vi "Calibrate In Ear.vi"(11 "State":T1) -> (0 "error out":errorcluster)   [LabVIEW 2020]
uses:
  epl-vi-lib/Utility VIs/Conversion VIs/Create Waveform Cluster (2D).vi
  Instance           1 24Saved   Calibrate In Ear .vi
  epl-vi-lib/Utility VIs/Type Defs/Speaker ring.ctl
  Type Defs/Cal Stimulus.ctl
  Type Defs/ACal-In Ear Parameters.ctl
  Type Defs/ACal-Multiband Parameters.ctl
  epl-vi-lib/Utility VIs/Math VIs/FFT x(t) to dB,Degrees (2D).vi
  epl-vi-lib/Utility VIs/File IO VIs/Configuration File Wrapper VIs/Config-Read Key (Boolean).vi
  cfts/LV Source/CFTS Main Panel SubVIs/CFTS-Experiment State.ctl
  epl-vi-lib/Utility VIs/Buttons/KCheckmarkBoolean 2.ctl
panel:
  in  "Speaker":T2
  in  "mic gain":dbl caption="Probe Mic Gain (dB)"
  in  "Stimulus":T3={"Min Freq (Hz)"=1000.0, "Max Freq (Hz)"=50000.0, "Freq Step (Hz)"=50.0, "Waveform"=0, "Attenuation (dB)"=30.0, "Sample Rate (Hz)"=100000.0} {"Waveform" items=["Chirp"]}
  out "Stimulus graph":cluster{i32, dbl, dbl[]}(graph)={0, 0.01, []}
  in  "Averages":i32=128
  in  "Return":bool
  in  "START":bool
  in  "STOP":bool
  out "Path":path
  in  "Data tab":enum32{"Raw", "Calibration"}(tab)
  out "Mic signals":cluster{"offset":dbl, "dx":dbl, "Y":dbl[][]}(graph)
  out "Mic mag":cluster{"offset":dbl, "dx":dbl, "Y":dbl[][]}(graph)
  out "Acquired":i32=256
  in  "Clear":bool
  in  "Load":bool
  in  "Show all":bool
  in  "Last N":bool
  out "ASTF":cluster{"Frequency":dbl[], "Frequency":dbl[]}[](graph)
  in  "Plot Max SPL":T4=TRUE
  in  "result":cluster{"Path":path, "error ":errorcluster}
  out "ASTF phase":cluster{"Frequency":dbl[], "Frequency":dbl[]}[](graph)
  out "Mic phase graph":cluster{"offset":dbl, "dx":dbl, "Y":dbl[][]}(graph)
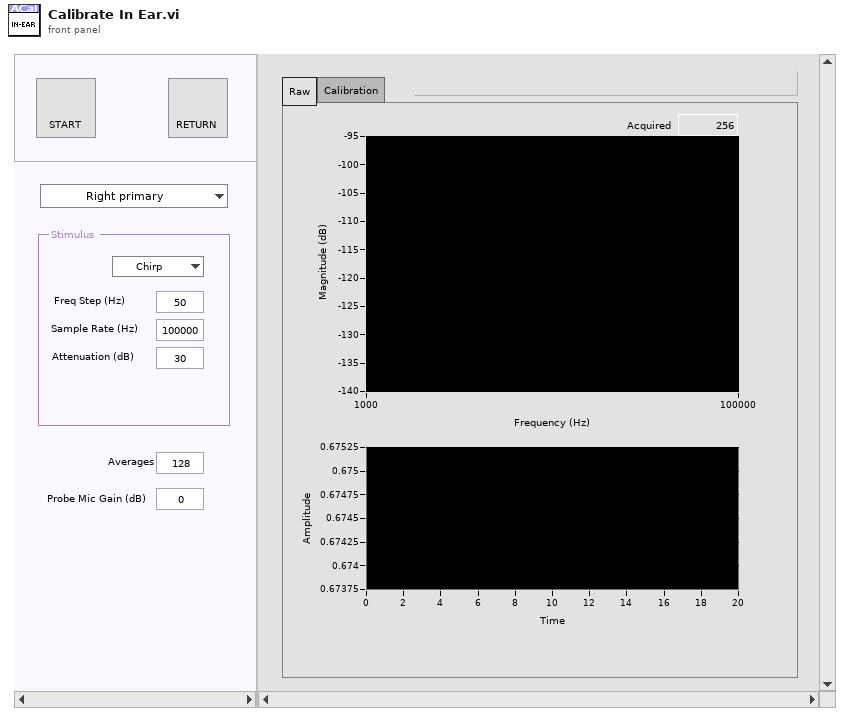
[diagram p1: front panel]
types:
  T1 = typedef "CFTS-Experiment State.ctl" = cluster{"Experimenter":string, "Number":u32, "Right":string, "Left":string, "Data Folder":path, "State File":path, "Version Info":string, "End Exposure Time":dbl, "Exposure Duration":string, "Run #":cluster{"CAP":i16, "ABR":i16, "DP":i16, "VsEP":i16, "MeasSeq":i16, "SubSeq":i16, "SFOAE":i16}}
  T2 = typedef "Speaker ring.ctl" = enum16{"Right primary", "Right secondary", "Left primary", "Left secondary"}
  T3 = cluster{"Min Freq (Hz)":dbl, "Max Freq (Hz)":dbl, "Freq Step (Hz)":dbl, "Waveform":u16, "Attenuation (dB)":dbl, "Sample Rate (Hz)":dbl}
  T4 = typedef "KCheckmarkBoolean 2.ctl" = bool
  T5 = typedef "ACal-In Ear Parameters.ctl" = cluster{"Speaker":T2, "Stimulus":T6, "Averages":i32, "Left gain":dbl, "Right gain":dbl, "plot max":bool, "smooth override":bool, "Weighted":T7, "Max Vmic":dbl}
  T6 = typedef "Cal Stimulus.ctl" = cluster{"Min Freq (Hz)":dbl, "Max Freq (Hz)":dbl, "Freq Step (Hz)":dbl, "Waveform":enum16{"Chirp", "Weighted"}, "Attenuation (dB)":dbl, "Sample Rate (Hz)":dbl}
  T7 = typedef "ACal-Multiband Parameters.ctl" = cluster{"Folder":path, "Fmin":dbl, "Fmax":dbl, "Max range":dbl, "WF":u16}
  T8 = typedef "Cal-Smoothing Parameters.ctl" = cluster{"Method":enum16{"None", "Moving average", "Loess"}, "MA":cluster{"Iterations":i32, "Length":i32}, "Loess":cluster{"Length":i32, "Type":enum16{"Linear", "Quadratic"}, "Robust":bool}}
  T9 = cluster{"new file path":path, "error out":errorcluster}
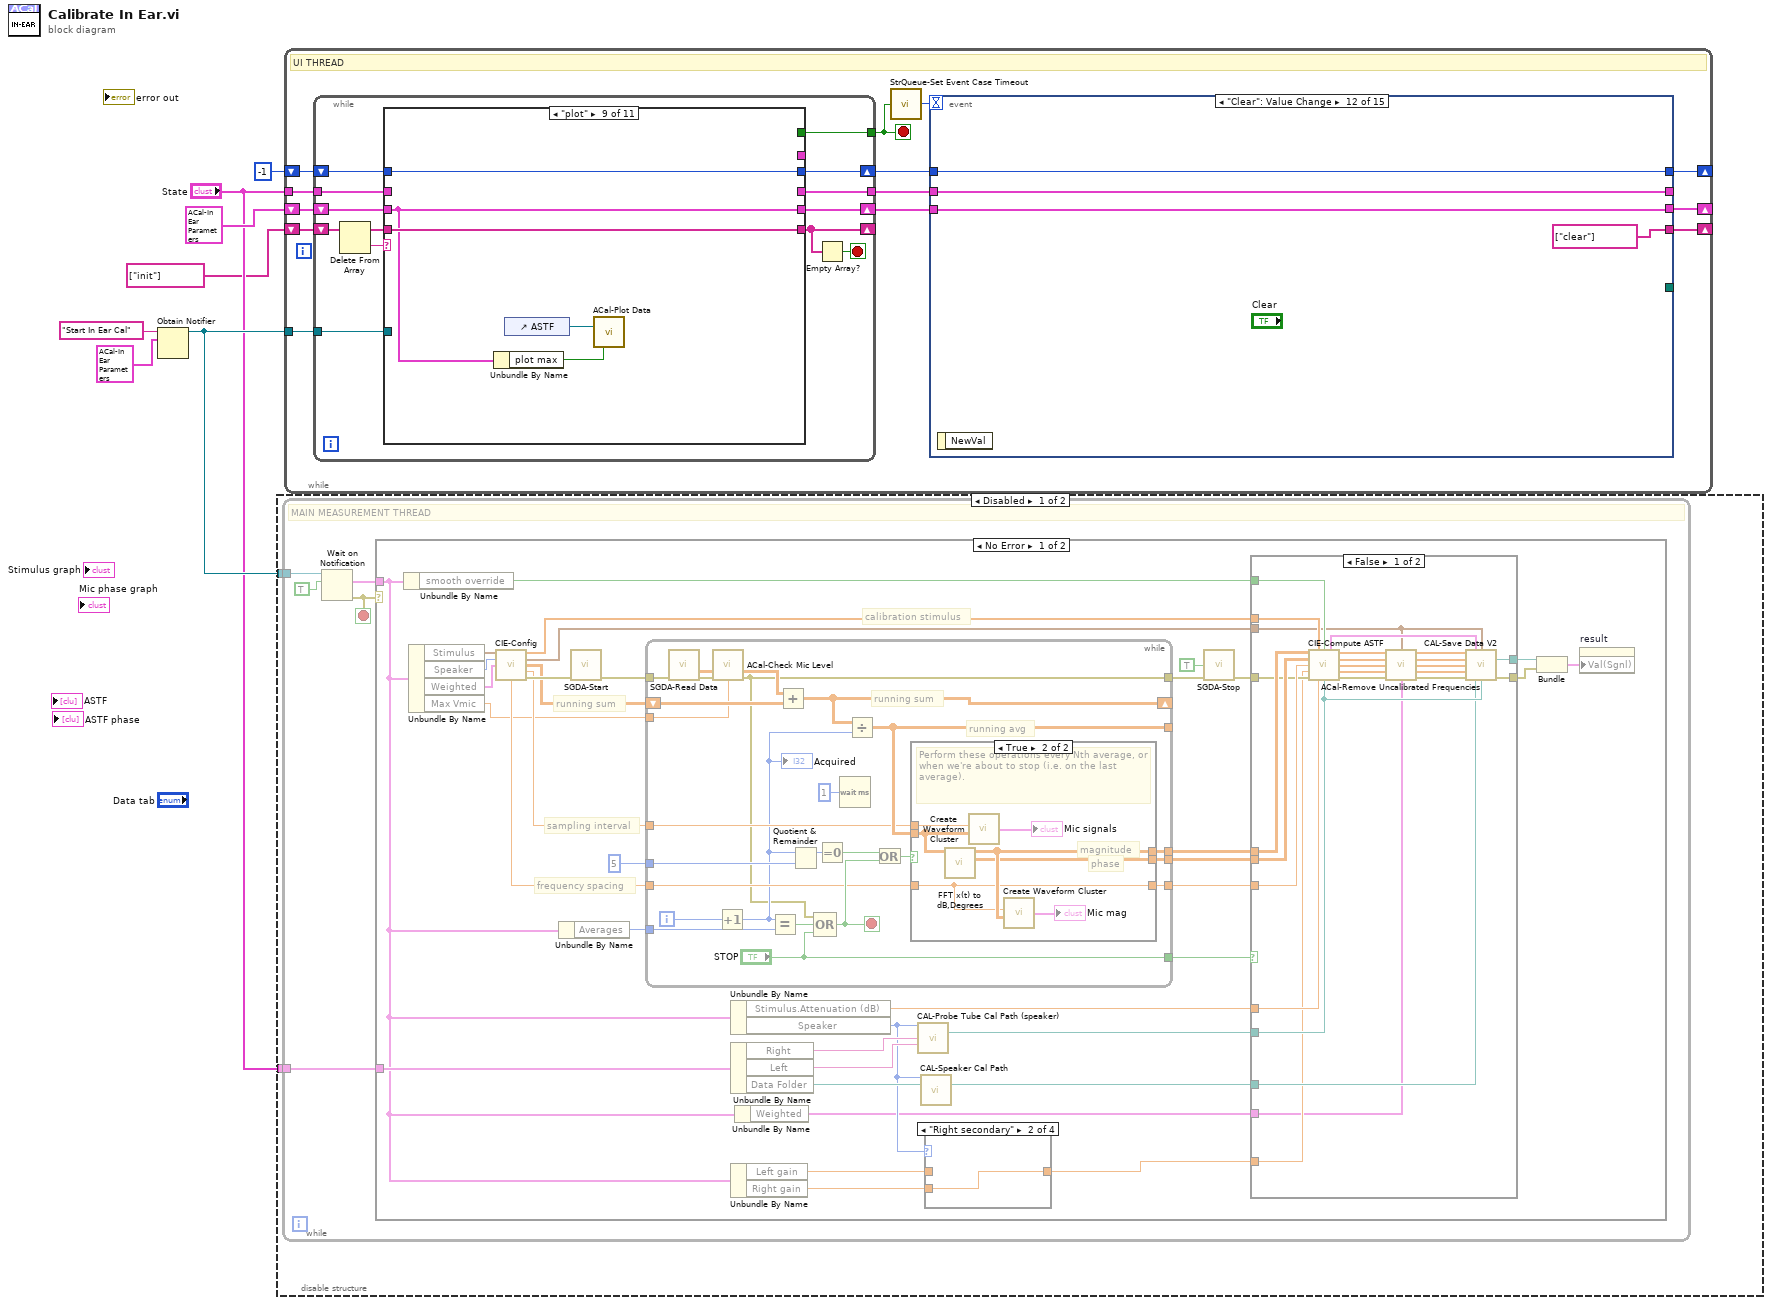
[diagram p0: block diagram]
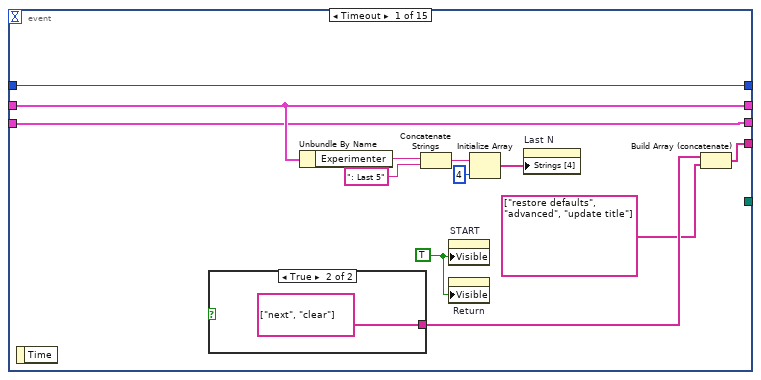
[diagram p9: hidden frame]
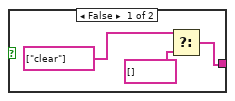
[diagram p10: hidden frame]
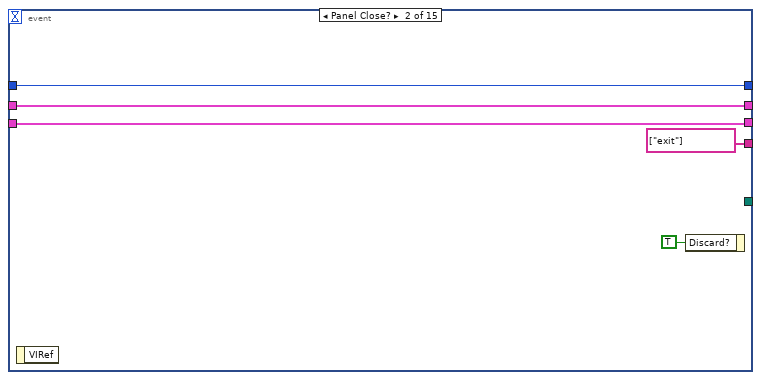
[diagram p11: hidden frame]
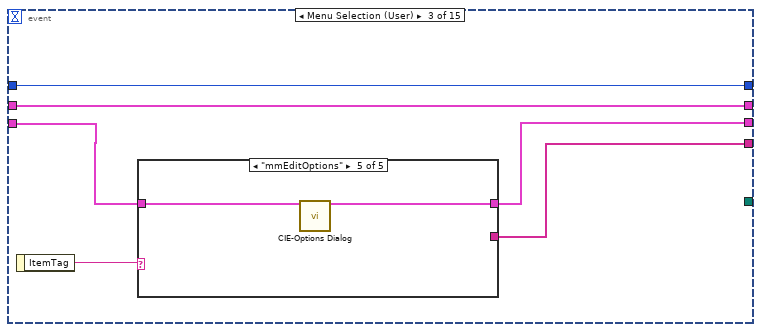
[diagram p12: hidden frame]
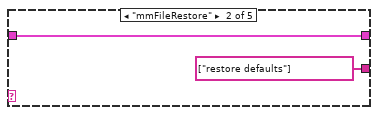
[diagram p14: hidden frame]
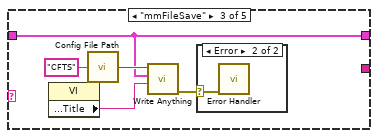
[diagram p15: hidden frame]
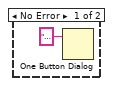
[diagram p16: hidden frame]
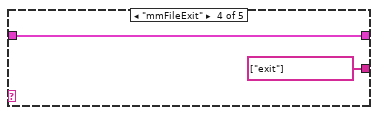
[diagram p17: hidden frame]
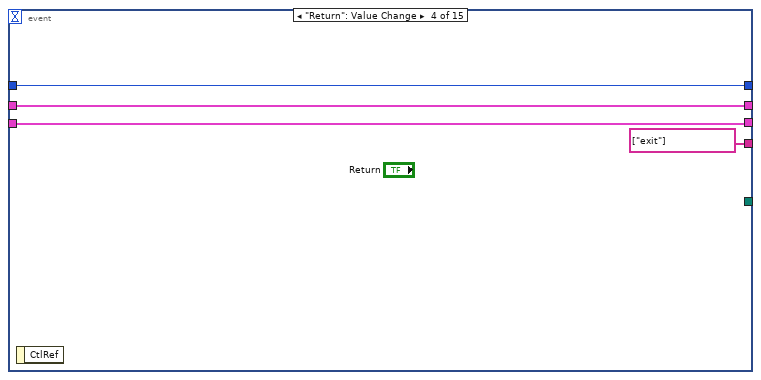
[diagram p18: hidden frame]
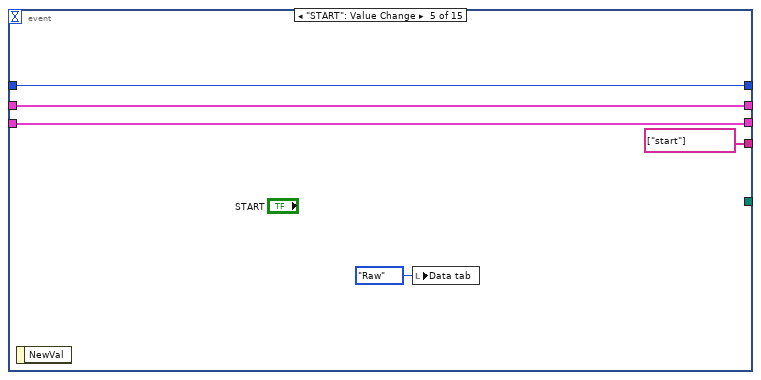
[diagram p19: hidden frame]
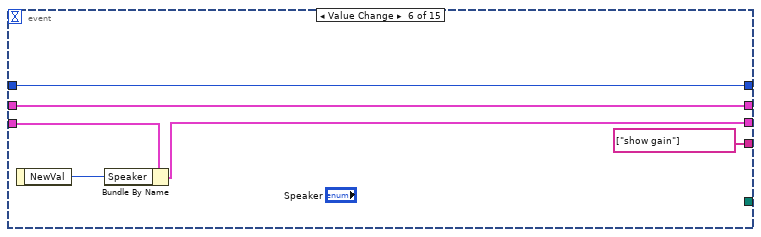
[diagram p20: hidden frame]
diagram:
  n1 = Obtain Notifier(name (unnamed)="Start In Ear Cal", notification data type=T5 {"Speaker"=enum."Right primary", "Stimulus"={"Min Freq (Hz)"=50.0, "Max Freq (Hz)"=50000.0, "Freq Step (Hz)"=50.0, "Waveform"=enum."Chirp", "Attenuation (dB)"=20.0, "Sample Rate (Hz)"=100000.0}, "Averages"=512, "Left gain"=40.0, "Right gain"=40.0, "plot max"=TRUE, "smooth override"=FALSE, "Weighted"={"Folder"=path "", "Fmin"=0.0, "Fmax"=0.0, "Max range"=0.0, "WF"=0}, "Max Vmic"=0.0} ("Params")) -> (notifier out=w7:refnum<notifier>)  [unwired: 2 in, 2 out]
  n2 = disable-structure shown="Disabled" {
    disable-tunnel: w7 -> [w9 _]
    disable-tunnel: "State" -> [w8 _]
    frame Disabled {
      n3 = while {
        tunnel: w9 -> [w14]
        tunnel: w8 -> [w12]
        stop <- w13 stop-if-true
        # "MAIN MEASUREMENT THREAD"
        n4 = Wait on Notification(notifier=w14, ignore previous (F)=TRUE) -> (notification=w11:T5, error out=w13:errorcluster)  [unwired: 2 in, 2 out]
        n5 = case shown="No Error" w13 {
          tunnel: w12 -> [w33 _]
          tunnel: w11 -> [w18 _]
          frame No Error {
            # "calibration stimulus"
            # "frequency spacing"
            # "sampling interval"
            # "running sum"
            n6 = Unbundle By Name(w18) -> ("smooth override"=w29:bool)
            n7 = Unbundle By Name(w18) -> ("Stimulus"=w32:T6, "Speaker"=w31:T2, "Weighted"=w19:T7, "Max Vmic"=w16:dbl)
            n8 = call "CIE-Config.vi"("Cal Stimulus"=w32, "Speaker"=w31, "Weighted"=w19) -> ("Stimulus"=w44:dbl[], "Cal Spec Out"=w35:T6, "Mic Avg"=w50:dbl[][], "dt (ms)"=w48:dbl, "df (Hz)"=w49:dbl, "error out"=w51:errorcluster)  [unwired: 6 in, 1 out]
            n9 = Unbundle By Name(w18) -> ("Averages"=w30:i32)
            n10 = call "SGDA-Start.vi"("error in (no error)"=w51) -> ("error out"=w43:errorcluster)  [unwired: 6 in]
            n11 = while {
              tunnel: w43 -> [w106]
              tunnel: [w82] -> w42
              tunnel: w30 -> [w103]
              shift-right: [w101] -> _
              shift-left: w50 -> [w102]
              tunnel: [w100] -> _
              tunnel: 5 -> [w99]
              tunnel: w49 -> [w94]
              tunnel: [w93] -> w47
              tunnel: [w92] -> w46
              tunnel: w48 -> [w91]
              tunnel: [w90] -> w45
              tunnel: ["STOP"] -> w27
              tunnel: w16 -> [w83]
              i -> [w105]
              stop <- w95 stop-if-true
              # "running avg"
              # "running sum"
              n12 = call "SGDA-Read Data.vi"("error in (no error)"=w106) -> ("AI Waveforms"=w85:dbl[][], "error out"=w86:errorcluster)  [unwired: 13 in]
              n13 = call "ACal-Check Mic Level.vi"("AI Waveforms in"=w85, "error in (no error)"=w86, "Max Vmic"=w83) -> ("AI Waveforms out"=w84:dbl[][], "error out"=w82:errorcluster)  [unwired: 11 in]
              n14 = Increment(x=w105) -> (x+1=w89:i32)
              "Acquired" <- w89
              n15 = Equal?(x=w89, y=w103) -> (x = y?=w104:bool)
              n16 = Add(x=w84, y=w102) -> (x+y=w101:dbl[][])
              n17 = Quotient & Remainder(x=w89, y=w99) -> (x-y*floor(x/y)=w98:i32)  [unwired: 1 out]
              n18 = Compound Arithmetic op=OR(w82, w104, "STOP") -> (w95:bool)
              n19 = Equal To 0?(x=w98) -> (x = 0?=w96:bool)
              n20 = Wait (ms)(milliseconds to wait=u32 1) -> ()  [unwired: 1 out]
              n21 = Divide(x=w101, y=w89) -> (x/y=w100:dbl[][])
              n22 = Or(x=w96, y=w95) -> (x .or. y?=w97:bool)
              n23 = case shown="True" w97 {
                tunnel: w100 -> [_ w110]
                tunnel: w94 -> [_ w107]
                tunnel: [_ w112] -> w93
                tunnel: [_ w111] -> w92
                tunnel: w91 -> [_ w109]
                tunnel: [_ w107] -> w90
                frame False {
                }
                frame True {
                  # "phase"
                  # "magnitude"
                  # "Perform these operations every Nth average, or when we're about to stop (i.e. on the last average)."
                  n24 = call-poly "FFT x(t) to dB,Degrees.vi"("X(t)"=w110) -> ("+Freq Phase of FFT (degrees)"=w111:dbl[][], "+Freq. Mag of FFT (dB rms)"=w112:dbl[][])  [unwired: 9 in]
                  n25 = call-poly "Create Waveform Cluster.vi"("dx"=w109, "Array"=w110) -> ("waveform cluster"=→"Mic signals":cluster{"offset":dbl, "dx":dbl, "Y":dbl[][]})  [unwired: 3 in]
                  n26 = call-poly "Create Waveform Cluster.vi"("dx"=w107, "Array"=w112) -> ("waveform cluster"=→"Mic mag":cluster{"offset":dbl, "dx":dbl, "Y":dbl[][]})  [unwired: 3 in]
                }
              }
            }
            n27 = Unbundle By Name(w18) -> ("Stimulus.Attenuation (dB)"=w28:dbl, "Speaker"=w26:T2)
            n28 = Unbundle By Name(w33) -> ("Right"=w40:string, "Left"=w39:string, "Data Folder"=w38:path)
            n29 = Unbundle By Name(w18) -> ("Left gain"=w25:dbl, "Right gain"=w23:dbl)
            n30 = Unbundle By Name(w18) -> ("Weighted"=w17:T7)
            n31 = call "CAL-Probe Tube Cal Path (speaker).vi"("Speaker"=w26, "Right"=w40, "Left"=w39) -> ("Probe Tube Cal Path"=w37:path)  [unwired: 11 in, 1 out]
            n32 = call "CAL-Speaker Cal Path.vi"("Speaker"=w26, "Data Folder"=w38) -> ("Cal Path"=w34:path)  [unwired: 12 in, 1 out]
            n33 = case shown="\"Right secondary\"" w26 {
              tunnel: w25 -> [_ _ w54 w55]
              tunnel: [w52 w53 w54 w55] -> w24
              tunnel: w23 -> [w52 w53 _ _]
              frame "Right primary", Default {
              }
              frame "Right secondary" {
              }
              frame "Left secondary" {
              }
              frame "Left primary" {
              }
            }
            n34 = call "SGDA-Stop.vi"("Clear ActiveX (F)"=TRUE, "error in (no error)"=w42) -> ("error out"=w36:errorcluster)  [unwired: 13 in]
            n35 = case shown="False" w27 {
              tunnel: w47 -> [w80 _]
              tunnel: w46 -> [w79 _]
              tunnel: w45 -> [w78 _]
              tunnel: w44 -> [w77 _]
              tunnel: w37 -> [w76 _]
              tunnel: w36 -> [w75 w81]
              tunnel: w35 -> [w57 _]
              tunnel: w34 -> [w73 _]
              tunnel: w29 -> [w72 _]
              tunnel: w28 -> [w71 _]
              tunnel: [w70 w81] -> w21
              tunnel: [w69 _] -> w22
              tunnel: w24 -> [w68 _]
              tunnel: w17 -> [w56 _]
              frame False {
                n36 = call "CIE-Compute ASTF.vi"("Mag"=w80, "Stimulus"=w77, "Force no smoothing?"=w72, "Phase"=w79, "df (Hz)"=w78, "Probe Mic Gain (dB)"=w68, "error in (no error)"=w75, "Attenuation (dB)"=w71, "Probe Tube Path"=w76) -> ("Smooth Params"=w74:T8, "ASTF Mag"=w59:dbl[], "ASTF Phase"=w60:dbl[], "Frequency"=w63:dbl[], "Unsmoothed Mag"=w64:dbl[], "error out"=w67:errorcluster)  [unwired: 1 in]
                n37 = call "ACal-Remove Uncalibrated Frequencies.vi"("ASTF Mag in"=w59, "Cal Spec Out"=w57, "ASTF Phase in"=w60, "Frequency in"=w63, "Unsmoothed Mag in"=w64, "error in (no error)"=w67, "Weighted"=w56) -> ("ASTF Mag out"=w58:dbl[], "ASTF Phase out"=w61:dbl[], "Frequency out"=w62:dbl[], "Unsmoothed Mag out"=w65:dbl[], "error out"=w66:errorcluster)  [unwired: 4 in]
                n38 = call "CAL-Save Data V2.vi"("Mag"=w58, "Smooth Params"=w74, "Cal Stimulus"=w57, "Phase"=w61, "Frequency"=w62, "Unsmoothed Mag"=w65, "error in (no error)"=w66, "path"=w73, "Probe Tube File"=w76) -> ("new file path"=w69:path, "error out"=w70:errorcluster)  [unwired: 5 in]
              }
              frame True {
              }
            }
            n39 = Bundle("new file path"=w22, "error out"=w21) -> (w20:T9)  [unwired: 1 in]
            n40 = property on="result" class="Clust (strict)"("Val(Sgnl)"=w20) -> ()  [unwired: 2 in, 2 out]
          }
          frame Error {
          }
        }
      }
    }
    frame Enabled {
    }
  }
  n41 = while {
    tunnel: w7 -> [w119]
    shift-right: [w114] -> _
    shift-left: -1 -> [w126]
    tunnel: "State" -> [w125]
    shift-right: [w115] -> _
    shift-left: T5 {"Speaker"=enum."Right primary", "Stimulus"={"Min Freq (Hz)"=50.0, "Max Freq (Hz)"=50000.0, "Freq Step (Hz)"=50.0, "Waveform"=enum."Chirp", "Attenuation (dB)"=20.0, "Sample Rate (Hz)"=100000.0}, "Averages"=512, "Left gain"=40.0, "Right gain"=40.0, "plot max"=TRUE, "smooth override"=FALSE, "Weighted"={"Folder"=path "C:/Data", "Fmin"=3000.0, "Fmax"=45000.0, "Max range"=25.0, "WF"=0}, "Max Vmic"=0.0} ("Params") -> [w124]
    shift-right: [w122] -> _
    shift-left: string[] ["init"] ("t") -> [w121]
    stop <- w117 stop-if-true
    # "UI THREAD"
    n42 = while {
      shift-right: [w261] -> w120
      shift-left: w124 -> [w262]
      shift-right: [w260] -> w123
      shift-left: w126 -> [w263]
      shift-right: [w256] -> _
      shift-left: w121 -> [w258]
      tunnel: w119 -> [w254]
      tunnel: [w253] -> w117
      tunnel: w125 -> [w252]
      tunnel: [w251] -> w116
      stop <- w255 stop-if-true
      n43 = Delete From Array(array=w258) -> (deleted portion=w257:string, array with subset deleted=w259:string[])  [unwired: 2 in]
      n44 = case shown="\"plot\"" w257 {
        tunnel: w263 -> [w266 w271 w277 w288 w299 w315 w331 w338 w345 w350 w361]
        tunnel: [w266 w271 w277 w288 w299 w315 w331 w338 w345 w350 w361] -> w260
        tunnel: w262 -> [w265 w270 w276 w287 w298 w310 w329 w336 w343 w346 w355]
        tunnel: [w265 w270 w276 w287 w298 w309 w329 w336 w343 w346 w354] -> w261
        tunnel: w259 -> [w264 w269 w275 w286 w297 w314 w330 w337 w344 w347 w353]
        tunnel: [w264 w269 w275 w286 w297 w308 w324 w337 w344 w347 w351] -> w256
        tunnel: w254 -> [_ _ w274 _ _ _ _ _ _ w348 _]
        tunnel: [_ _ TRUE _ _ _ _ _ _ _ w358] -> w253
        tunnel: w252 -> [_ _ w272 w279 _ _ _ _ _ _ _]
        tunnel: [_ _ _ _ w293 _ _ _ _ _ w352] -> _
        tunnel: [_ _ w272 _ _ _ _ _ _ _ _] -> w251
        frame "", Default {
        }
        frame "clear" {
          w268 = cluster{"Frequency":dbl[], "Frequency":dbl[]}[] [] ("ASTF mag")
          n45 = property on="ASTF phase" class="XYGraph (strict)"("Value"=w268) -> ()  [unwired: 2 in, 2 out]
          n46 = property on="ASTF" class="XYGraph (strict)"("Legend Visible"=FALSE ("Legend:Visible"), "Value"=w268) -> ()  [unwired: 2 in, 2 out]
        }
        frame "exit" {
          n47 = Release Notifier(notifier=w274) -> ()  [unwired: 2 in, 3 out]
        }
        frame "update title" {
          n48 = Unbundle By Name(w279) -> ("Experimenter"=w278:string)
          n49 = control-ref of="This VI"() -> (w280:refnum<vi>)
          n50 = call "CFTS-Is Advanced User.vi"("Experimenter"=w278) -> ("Advanced user"=w283:bool)
          n51 = call "Config File Path.vi"("AppName"="CFTS") -> ("Default config file name"=w281:path)
          n52 = Select(t=w278, s=w283, f="") -> (s? t:f=w285:string)
          n53 = call "Append User ID To Section Label.vi"("VI reference"=w280, "Path (dialog)"=w281, "User"=w285) -> ()  [unwired: 9 in, 4 out]
        }
        frame "advanced" {
          n54 = call "PXI-Connections File Path.vi"() -> ("Path"=w294:path)  [unwired: 1 in]
          n55 = call-poly "Config-Read Key.vi"("configuration file path"=w294, "key"="Advanced in-ear", "default"=FALSE) -> ("value"=w292:bool)  [unwired: 9 in, 3 out]
          n56 = case shown="True" w292 {
            tunnel: "Chirp" ("key") -> [w301 w304]
            tunnel: "Weighted" ("key") -> [_ w303]
            tunnel: [w300 w302] -> w289
            frame False {
              n57 = Build Array(w301) -> (w300:string[])
            }
            frame True {
              n58 = Build Array(w304, w303) -> (w302:string[])
            }
          }
          n59 = Bundle By Name("advanced"=w292) -> (w293:cluster{})  [unwired: 1 in]
          n60 = property on="Waveform" class="Ring (strict)"("Strings []"=w289) -> ()  [unwired: 2 in, 2 out]
        }
        frame "restore defaults" {
          n61 = property class="VI"() -> ("Front Panel.Title"=w306:string)  [unwired: 2 in, 2 out]
          n62 = call "Config File Path.vi"("AppName"="CFTS") -> ("Default config file name"=w305:path)
          n63 = call "Read Anything.vi"("Type of Anything"=w310, "Section Name (Name of \"Type of Anything\")"=w306, "Path (dialog)"=w305) -> ("Found?"=w312:bool, "Anything"=w311:variant)  [unwired: 6 in, 1 out]
          n64 = case shown="False" w312 {
            tunnel: w311 -> [_ w321]
            tunnel: w310 -> [w318 w320]
            tunnel: [w317 w319] -> w309
            tunnel: w306 -> [w316 _]
            frame False {
              n65 = call "ACal-Update In Ear Parameters.vi"("Params in"=w318, "Section"=w316) -> ("Params out"=w317:T5)  [unwired: 13 in]
            }
            frame True {
              n66 = Variant To Data(type=w320, Variant=w321) -> (data=w319:T5)  [unwired: 1 in, 1 out]
            }
          }
          n67 = Build Array (concatenate)(w314, "show params") -> (w308:string[])
        }
        frame "show params" {
          n68 = Unbundle By Name(w329) -> ("Speaker"=w328:T2, "Stimulus"=w327:T6, "Averages"=w326:i32, "plot max"=w325:bool)
          n69 = local write "Speaker"(w328) -> ()
          n70 = local write "Stimulus"(w327) -> ()
          n71 = local write "Averages"(w326) -> ()
          n72 = local write "Plot Max SPL"(w325) -> ()
          n73 = Build Array (concatenate)(w330, "show gain", "show wf") -> (w324:string[])
        }
        frame "show gain" {
          n74 = Unbundle By Name(w336) -> ("Speaker"=w334:T2, "Left gain"=w333:dbl, "Right gain"=w332:dbl)
          n75 = case shown="\"Right primary\", \"Right secondary\"" w334 {
            tunnel: w333 -> [w339 _]
            tunnel: w332 -> [_ w340]
            tunnel: [w339 w340] -> w335
            frame "Left primary", Default {
            }
            frame "Right primary", "Right secondary" {
            }
          }
          n76 = local write "mic gain"(w335) -> ()
        }
        frame "plot" {
          n77 = Unbundle By Name(w343) -> ("plot max"=w342:bool)
          n78 = control-ref of="ASTF"() -> (w341:refnum<vi>)
          n79 = call "ACal-Plot Data.vi"("Mag graph"=w341, "Plot max"=w342) -> ()  [unwired: 12 in, 2 out]
        }
        frame "start" {
          w349 = FALSE
          n80 = Send Notification(notification=w346, notifier=w348) -> ()  [unwired: 1 in, 2 out]
          n81 = property on="Return" class="Bool"("Visible"=w349) -> ()  [unwired: 2 in, 2 out]
          n82 = property on="START" class="Bool"("Visible"=w349) -> ()  [unwired: 2 in, 2 out]
        }
        frame "next" {
          w357 = T2[] [enum."Right primary", enum."Right secondary", enum."Left primary", enum."Left secondary"] items=["Right primary", "Right secondary", "Left primary", "Left secondary"]
          n83 = Unbundle By Name() -> ()  [unwired: 1 in, 1 out]
          n84 = Array Size(array=w357) -> (size(s)=w360:i32)
          n85 = Increment() -> (x+1=w356:dbl)  [unwired: 1 in]
          n86 = Less?(x=w356, y=w360) -> (x < y?=w359:bool)
          n87 = case shown="True" w359 {
            tunnel: [TRUE _] -> w358
            tunnel: w357 -> [_ w371]
            tunnel: w356 -> [_ w367]
            tunnel: w355 -> [w363 w370]
            tunnel: [w363 w368] -> w354
            tunnel: [w362 string[] ["start"]] -> w351
            tunnel: w353 -> [w362 _]
            tunnel: [_ w366] -> w352
            frame False {
            }
            frame True {
              n88 = Index Array(array=w371, index=w367) -> (element=w369:T2)
              n89 = Bundle By Name(cluster=w370, "Speaker"=w369) -> (w368:T5)
              n90 = local write "Speaker"(w369) -> ()
              n91 = Bundle By Name("next"=w367) -> (w366:cluster{})  [unwired: 1 in]
            }
          }
        }
      }
      n92 = Empty Array?(array=w256) -> (empty?=w255:bool)
    }
    n93 = call "StrQueue-Set Event Case Timeout.vi"("Quit"=w117) -> ("timeout"=w118:i32)  [unwired: 14 in]
    n94 = event shown="[11] \"Clear\": Value Change" {
      selector: _ -> [_ _ _ _ _ _ _ _ _ _ _ _ _ _ _]
      dyn-events: _ -> [_ _ _ _ _ _ _ _ _ _ _ _ _ _ _]
      timeout: w118 -> [_ _ _ _ _ _ _ _ _ _ _ _ _ _ _]
      tunnel: w123 -> [w132 w146 w153 w171 w176 w182 w186 w191 w198 w209 w218 w228 w233 w244 w249]
      tunnel: [w132 w146 w153 w171 w176 w182 w186 w191 w198 w209 w218 w228 w233 w244 w249] -> w114
      tunnel: w120 -> [w127 w143 w149 w169 w173 w179 w185 w190 w194 w206 w210 w225 w232 w242 w246]
      tunnel: [w127 w143 w151 w169 w173 w178 w184 w189 w193 w205 w210 w225 w232 w242 w246] -> w115
      tunnel: [w130 string[] ["exit"] w150 string[] ["exit"] string[] ["start"] string[] ["show gain"] _ _ _ _ w214 string[] ["clear"] w230 _ _] -> w122
      tunnel: [w128 w144 w148 w168 w172 w177 w183 w188 w195 w207 w211 w226 w229 w241 w247] -> _
      tunnel: [_ _ _ _ _ _ _ _ _ _ w216 _ w231 _ _] -> _
      tunnel: w116 -> [w128 w144 w148 w168 w172 w177 w183 w188 w195 w207 w211 w226 w229 w241 w247]
      event Timeout {
        w138 = TRUE ("Visible")
        n95 = event-data() -> ()  [unwired: 1 in, 1 out]
        n96 = case shown="True" {
          selector: _ -> [_ _]
          tunnel: [w140 string[] ["next", "clear"]] -> w131
          frame False {
            n97 = Select(t=string[] ["clear"], f=string[] []) -> (s? t:f=w140:string[])  [unwired: 1 in]
          }
          frame True {
          }
        }
        n98 = Unbundle By Name(w128) -> ("Experimenter"=w137:string)
        n99 = Concatenate Strings(w137, ": Last 5" ("string")) -> (w135:string)
        n100 = property on="START" class="Bool"("Visible"=w138) -> ()  [unwired: 2 in, 2 out]
        n101 = property on="Return" class="Bool"("Visible"=w138) -> ()  [unwired: 2 in, 2 out]
        n102 = Initialize Array(w135, 4 ("dimension size")) -> (w133:string[])
        n103 = property on="Last N" class="Bool"("Strings [4]"=w133) -> ()  [unwired: 2 in, 2 out]
        n104 = Build Array (concatenate)(w131, string[] ["restore defaults", "advanced", "update title"]) -> (w130:string[])
      }
      event Panel Close? {
        n105 = event-data() -> ()  [unwired: 1 in, 1 out]
        n106 = event-data("Discard?"=TRUE) -> ()  [unwired: 1 in, 1 out]
      }
      event Menu Selection (User) {
        n107 = event-data() -> ("ItemTag"=w152:string)  [unwired: 1 in]
        n108 = case shown="\"mmEditOptions\"" w152 {
          tunnel: w149 -> [w154 w156 w159 w165 w167]
          tunnel: [w154 w156 w159 w165 w166] -> w151
          tunnel: [_ string[] ["restore defaults"] _ string[] ["exit"] _] -> w150
          frame "", Default {
          }
          frame "mmFileRestore" {
          }
          frame "mmFileSave" {
            n109 = property class="VI"() -> ("Front Panel.Title"=w158:string)  [unwired: 2 in, 2 out]
            n110 = call "Config File Path.vi"("AppName"="CFTS") -> ("Default config file name"=w160:path)
            n111 = call "Write Anything.vi"("Section Name (Name of \"Anything\")"=w158, "Anything"=w159, "Path (dialog)"=w160) -> ("Error Out"=w157:errorcluster)  [unwired: 7 in, 1 out]
            n112 = case shown="Error" w157 {
              selector: w157 -> [_ w163]
              frame No Error {
                n113 = One Button Dialog(message="Defaults saved.") -> ()  [unwired: 1 in, 1 out]
              }
              frame Error {
                n114 = call "Error Handler.vi"("error in (no error)"=w163) -> ()  [unwired: 13 in, 2 out]
              }
            }
          }
          frame "mmFileExit" {
          }
          frame "mmEditOptions" {
            n115 = call "CIE-Options Dialog.vi"("Override smoothing"=w167) -> ("Override Out"=w166:T5)  [unwired: 13 in, 1 out]
          }
        }
      }
      event "Return": Value Change {
        n116 = event-data() -> ()  [unwired: 1 in, 1 out]
      }
      event "START": Value Change {
        n117 = event-data() -> ()  [unwired: 1 in, 1 out]
        n118 = local write "Data tab"(enum32{"Raw", "Calibration"}."Raw" ("Data tab")) -> ()
      }
      event Value Change {
        n119 = event-data() -> ("NewVal"=w180:T2)  [unwired: 1 in]
        n120 = Bundle By Name(cluster=w179, "Speaker"=w180) -> (w178:T5)
      }
      event "Stimulus": Value Change {
        n121 = event-data() -> ()  [unwired: 1 in, 1 out]
        n122 = Bundle By Name(cluster=w185, "Stimulus"="Stimulus") -> (w184:T5)
      }
      event "Averages": Value Change {
        n123 = event-data() -> ()  [unwired: 1 in, 1 out]
        n124 = Bundle By Name(cluster=w190, "Averages"="Averages") -> (w189:T5)
      }
      event "mic gain": Value Change {
        n125 = event-data() -> ()  [unwired: 1 in, 1 out]
        n126 = Unbundle By Name(w194) -> ("Speaker"=w196:T2)
        n127 = case shown="\"Left primary\", Default" w196 {
          tunnel: [w201 w204] -> w193
          tunnel: "mic gain" -> [w200 w203]
          tunnel: w194 -> [w199 w202]
          frame "Left primary", Default {
            n128 = Bundle By Name(cluster=w199, "Left gain"=w200) -> (w201:T5)
          }
          frame "Right primary", "Right secondary" {
            n129 = Bundle By Name(cluster=w202, "Right gain"=w203) -> (w204:T5)
          }
        }
      }
      event Value Change {
        n130 = event-data() -> ()  [unwired: 1 in, 1 out]
        n131 = Bundle By Name(cluster=w206, "plot max"="Plot Max SPL") -> (w205:T5)
      }
      event "result": Value Change {
        w215 = TRUE
        n132 = event-data() -> ("NewVal.Path"=w217:path, "NewVal.error"=w213:errorcluster)  [unwired: 1 in]
        n133 = call "Beeper.vi"() -> ()  [unwired: 5 in, 1 out]
        n134 = case shown="No Error" w213 {
          selector: w213 -> [_ w224]
          tunnel: w217 -> [w223 _]
          tunnel: [w223 _] -> w216
          tunnel: [w220 _] -> w214
          frame No Error {
            n135 = Empty String/Path?(string/path=w223) -> (empty?=w222:bool)
            n136 = Select(t=string[] [], s=w222, f=string[] ["plot"]) -> (s? t:f=w220:string[])
            "Path" <- w223
          }
          frame Error {
            n137 = call "Error Handler.vi"("error in (no error)"=w224) -> ()  [unwired: 13 in, 2 out]
          }
        }
        n138 = local write "Data tab"(enum32{"Raw", "Calibration"}."Calibration" ("Data tab")) -> ()
        n139 = property on="START" class="Bool"("Visible"=w215) -> ()  [unwired: 2 in, 2 out]
        n140 = property on="Return" class="Bool"("Visible"=w215) -> ()  [unwired: 2 in, 2 out]
      }
      event "Clear": Value Change {
        n141 = event-data() -> ()  [unwired: 1 in, 1 out]
      }
      event "Load": Value Change {
        n142 = event-data() -> ()  [unwired: 1 in, 1 out]
        n143 = Unbundle By Name(w232) -> ()  [unwired: 1 out]
        n144 = call "File Dialog"("pattern (all files)"="*.calib", "pattern label"="Calibration files") -> ("selected path"=w238:path, "cancelled"=w237:bool, "error out"=w236:errorcluster)  [unwired: 10 in, 1 out]
        n145 = case shown="False" w237 {
          tunnel: w238 -> [w240 _]
          tunnel: w236 -> [_ _]
          tunnel: [w240 _] -> w231
          tunnel: [string[] ["plot"] _] -> w230
          frame False {
          }
          frame True {
          }
        }
      }
      event "Show all": Value Change {
        n146 = event-data() -> ()  [unwired: 1 in, 1 out]
        n147 = Unbundle By Name() -> ()  [unwired: 1 in, 1 out]
        n148 = Unbundle By Name(w242) -> ()  [unwired: 1 out]
        n149 = control-ref of="ASTF"() -> (w243:refnum<vi>)
        n150 = call "CAL-Show all.vi"("Mag graph"=w243) -> ("error out"=w245:errorcluster)  [unwired: 13 in, 1 out]
        n151 = call "Error Handler.vi"("error in (no error)"=w245) -> ()  [unwired: 13 in, 2 out]
      }
      event "Last N": Value Change {
        n152 = event-data() -> ()  [unwired: 1 in, 1 out]
        n153 = Unbundle By Name() -> ()  [unwired: 1 in, 2 out]
        n154 = control-ref of="ASTF"() -> (w248:refnum<vi>)
        n155 = call "CAL-Show Last N.vi"("Mag graph"=w248) -> ("error out"=w250:errorcluster)  [unwired: 14 in]
        n156 = call <vilib>:"Simple Error Handler.vi"("error in (no error)"=w250) -> ()  [unwired: 4 in, 5 out]
      }
    }
  }
